vi "3 Gaussians Fit Guess Parameters.vi"(9 "Cursor X Array":dbl[](array[numeric]), 10 "Y Array":dbl[](array[numeric]), 11 "X Array":dbl[](array[numeric])) -> (1 "Guess Parameters Array":dbl[](array[numeric]), 2 "Y Array dup":dbl[](array[numeric]), 3 "X Array dup":dbl[](array[numeric]))   [LabVIEW 2019]
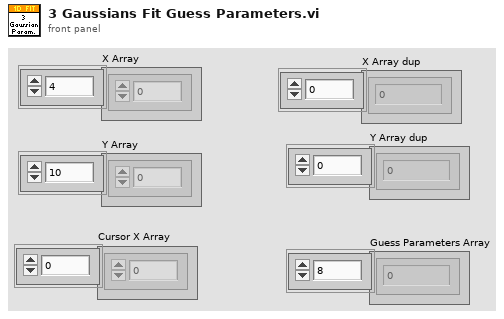
[diagram p1: front panel]
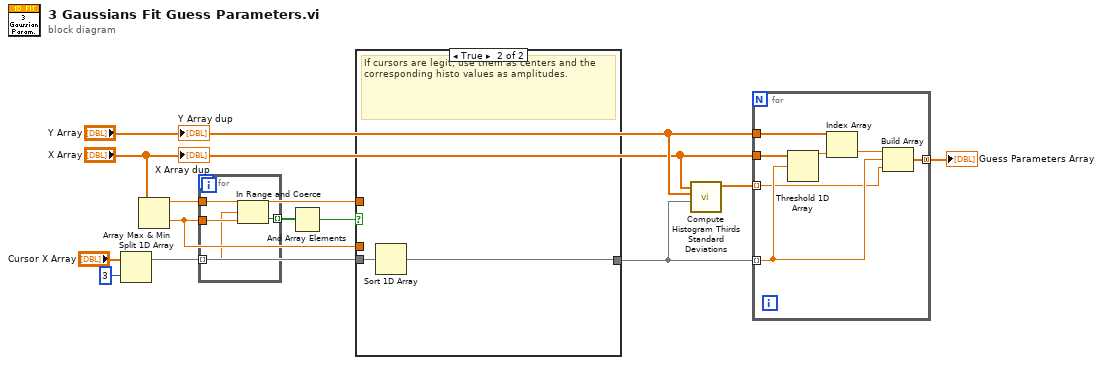
[diagram p0: block diagram]
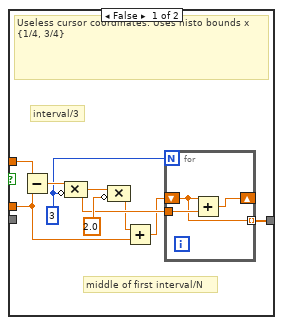
[diagram p2: hidden frame]
diagram:
  n1 = Split 1D Array(array="Cursor X Array", index=3) -> (first subarray=w1:dbl[])  [unwired: 1 out]
  n2 = Array Max & Min(array="X Array") -> (max value=w9:dbl, min value=w8:dbl)  [unwired: 2 out]
  n3 = for {
    tunnel: w9 -> [w16]
    tunnel: w8 -> [w15]
    tunnel: w1 -> [w14] mode=indexing
    tunnel: [w13] -> w12 mode=indexing
    n4 = In Range and Coerce(upper limit=w16, x=w14, lower limit=w15) -> (In Range?=w13:bool)  [unwired: 1 out]
  }
  n5 = And Array Elements(Boolean array=w12) -> (logical AND=w7:bool)
  n6 = case shown="True" w7 {
    tunnel: w1 -> [_ w30]
    tunnel: [w21 w29] -> w4
    tunnel: w9 -> [w25 _]
    tunnel: w8 -> [w19 _]
    frame False {
      w17 = 3 ("value")
      # "middle of first interval/N"
      # "interval/3"
      # "Useless cursor coordinates. Uses histo bounds x {1/4, 3/4}"
      n7 = Subtract(x=w25, y=w19) -> (x-y=w24:dbl)
      n8 = Compound Arithmetic op=MULTIPLY(w24, invert w17) -> (w22:dbl)
      n9 = Compound Arithmetic op=MULTIPLY(w22, invert 2.0 ("value")) -> (w20:dbl)
      n10 = Add(x=w20, y=w19) -> (x+y=w18:dbl)
      n11 = for {
        N: w17 -> [_]
        shift-right: [w28] -> _
        shift-left: w18 -> [w26]
        tunnel: w22 -> [w27]
        tunnel: [w26] -> w21 mode=indexing
        n12 = Add(x=w26, y=w27) -> (x+y=w28:dbl)
      }
    }
    frame True {
      # "If cursors are legit, use them as centers and the corresponding histo values as amplitudes."
      n13 = Sort 1D Array(array=w30) -> (sorted array=w29:dbl[])
    }
  }
  n14 = call "Compute Histogram Thirds Standard Deviations.vi"("Peak Positions"=w4, "Y Array"="Y Array", "X Array"="X Array") -> ("SDV Array"=w3:dbl[])  [unwired: 7 in, 1 out]
  n15 = for {
    tunnel: "X Array" -> [w36]
    tunnel: "Y Array" -> [w35]
    tunnel: w4 -> [w33] mode=indexing
    tunnel: [w32] -> w10 mode=concatenating
    tunnel: w3 -> [w31] mode=indexing
    n16 = Threshold 1D Array(2:w33, 3:w36) -> (0:w37:dbl)  [unwired: 1 in]
    n17 = Index Array(array=w35, index=w37) -> (element=w34:dbl)
    n18 = Build Array(w34, w33, w31) -> (w32:dbl[])
  }
  "Guess Parameters Array" <- w10
  "X Array dup" <- "X Array"
  "Y Array dup" <- "Y Array"
